vi "Main.vi"() -> ()   [LabVIEW 2021]
uses:
  DAQmxParams.ctl
  <vilib>/DAQmx/write.llb/DAQmx Write (Analog Wfm 1Chan NSamp).vi
  <vilib>/DAQmx/read.llb/DAQmx Read (Analog 1D Wfm NChan NSamp).vi
  <vilib>/DAQmx/create/channels.llb/DAQmx Create Channel (AO-Voltage-Basic).vi
  <vilib>/measure/matone.llb/Extract Single Tone Information 1 Chan.vi
  <vilib>/DAQmx/configure/timing.llb/DAQmx Timing (Sample Clock).vi
  <vilib>/DAQmx/miscellaneous.llb/DAQmx Fill In Error Info.vi
  <vilib>/DAQmx/create/channels.llb/DAQmx Create Channel (AI-Voltage-Basic).vi
  <vilib>/DAQmx/configure/trigger.llb/DAQmx Start Trigger (Analog Edge).vi
  <vilib>/measure/matone.llb/Extract Single Tone Information N Chan.vi
  <vilib>/measure/NI_MABase.lvlib
  <vilib>/measure/NI_MAPro.lvlib
panel:
  in  "Folder Path":path
  in  "Interval (ms)":dbl
  in  "Analyze Frequency":bool
  in  "Save analisys to file":bool
  in  "Stop frequency (Hz)":dbl
  in  "Start frequency (Hz)":dbl
  out "Phase":T1(graph)
  out "Amplitude":T2(graph)
  in  "Simulation":bool
  in  "V_out channel":tag
  in  "N samples/write":i32(slide)=1 min=1 scale=0.0..1000.0
  in  "Samples/s":i32=1 min=1
  in  "Trigger Channel":string(combo)
  in  "Function gen. 2":bool
  in  "Function gen. 1":bool
  in  "Frequency 2 (Hz)":dbl(knob) scale=0.0..10000.0
  in  "Amplitude 2 (V)":dbl(slide) scale=0.0..10.0
  in  "Frequency 1 (Hz)":dbl(knob) scale=0.0..10000.0
  in  "Amplitude 1 (V)":dbl(slide) scale=0.0..10.0
  in  "V_W Aq":bool
  in  "V_T Aq":bool
  in  "V_S Aq":bool
  in  "V_W":tag
  in  "V_T":tag
  in  "V_S":tag
  in  "Save acquisition to file":bool
  in  "DAQ Params":T3 {"Trigger Slope" items=["Rising"=10280, "Falling"=10171, "None"=0]; "Trigger Level" scale=-10.0..10.0}
  in  "Acquisition":bool
  out "Acquisition graph":waveform(dbl)[](graph)
  # "Function generator"
  # "Data acquisition"
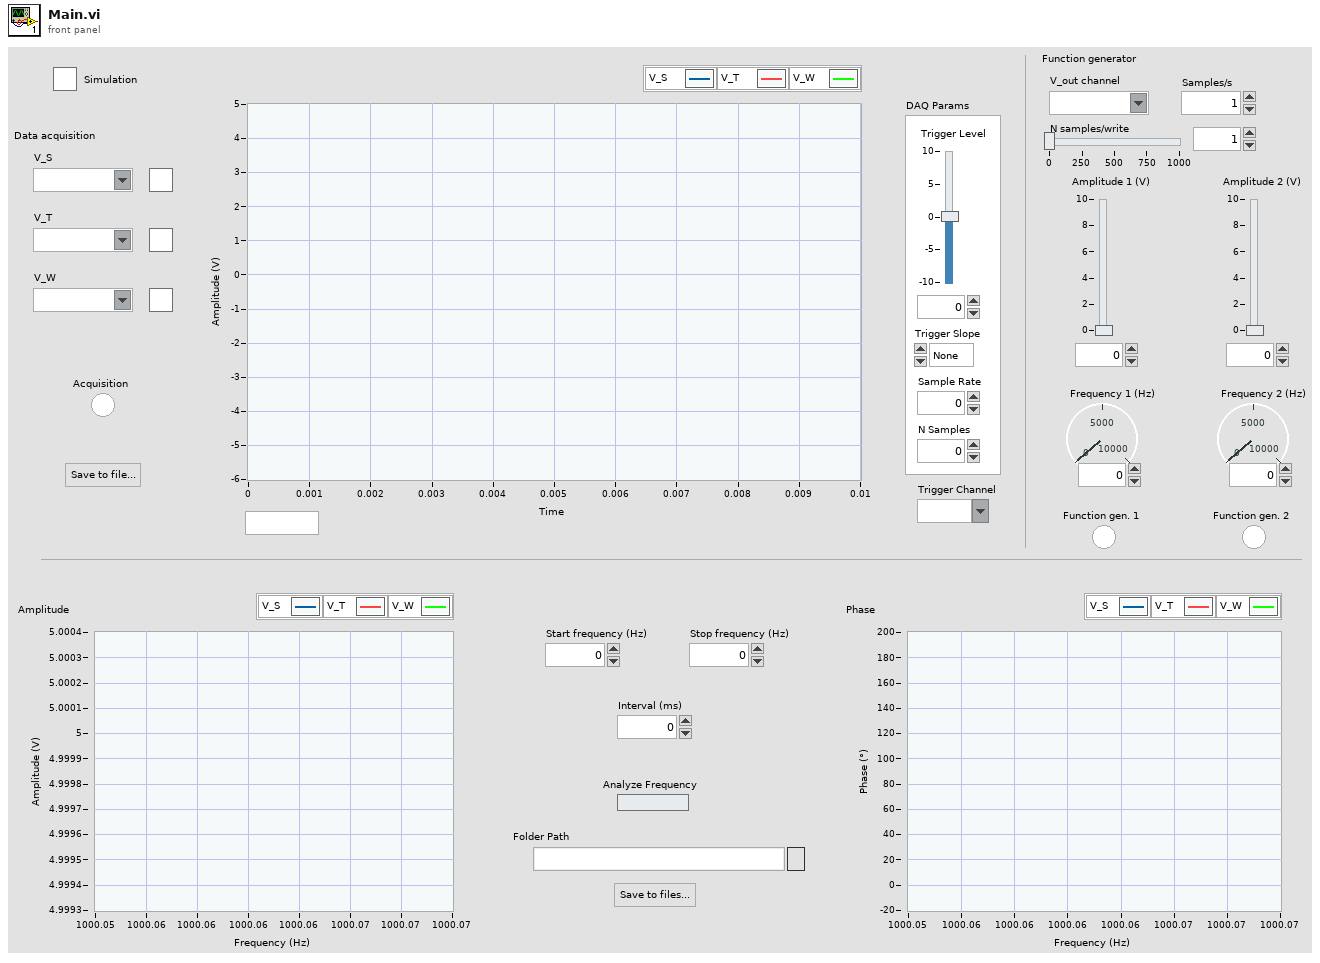
[diagram p1: front panel]
types:
  T1 = cluster{"detected frequencies":dbl[], "detected phases (deg)":dbl[]}[]
  T2 = cluster{"detected frequencies":dbl[], "detected amplitudes":dbl[]}[]
  T3 = typedef "DAQmxParams.ctl" = cluster{"Trigger Level":dbl, "Trigger Slope":i32, "Sample Rate":dbl, "N Samples":i32}
  T4 = enum8{"Enabled", "Disabled", "Disabled and Grayed Out"}
  T5 = enum16{"Sine Wave", "Triangle Wave", "Square Wave", "Sawtooth Wave"}
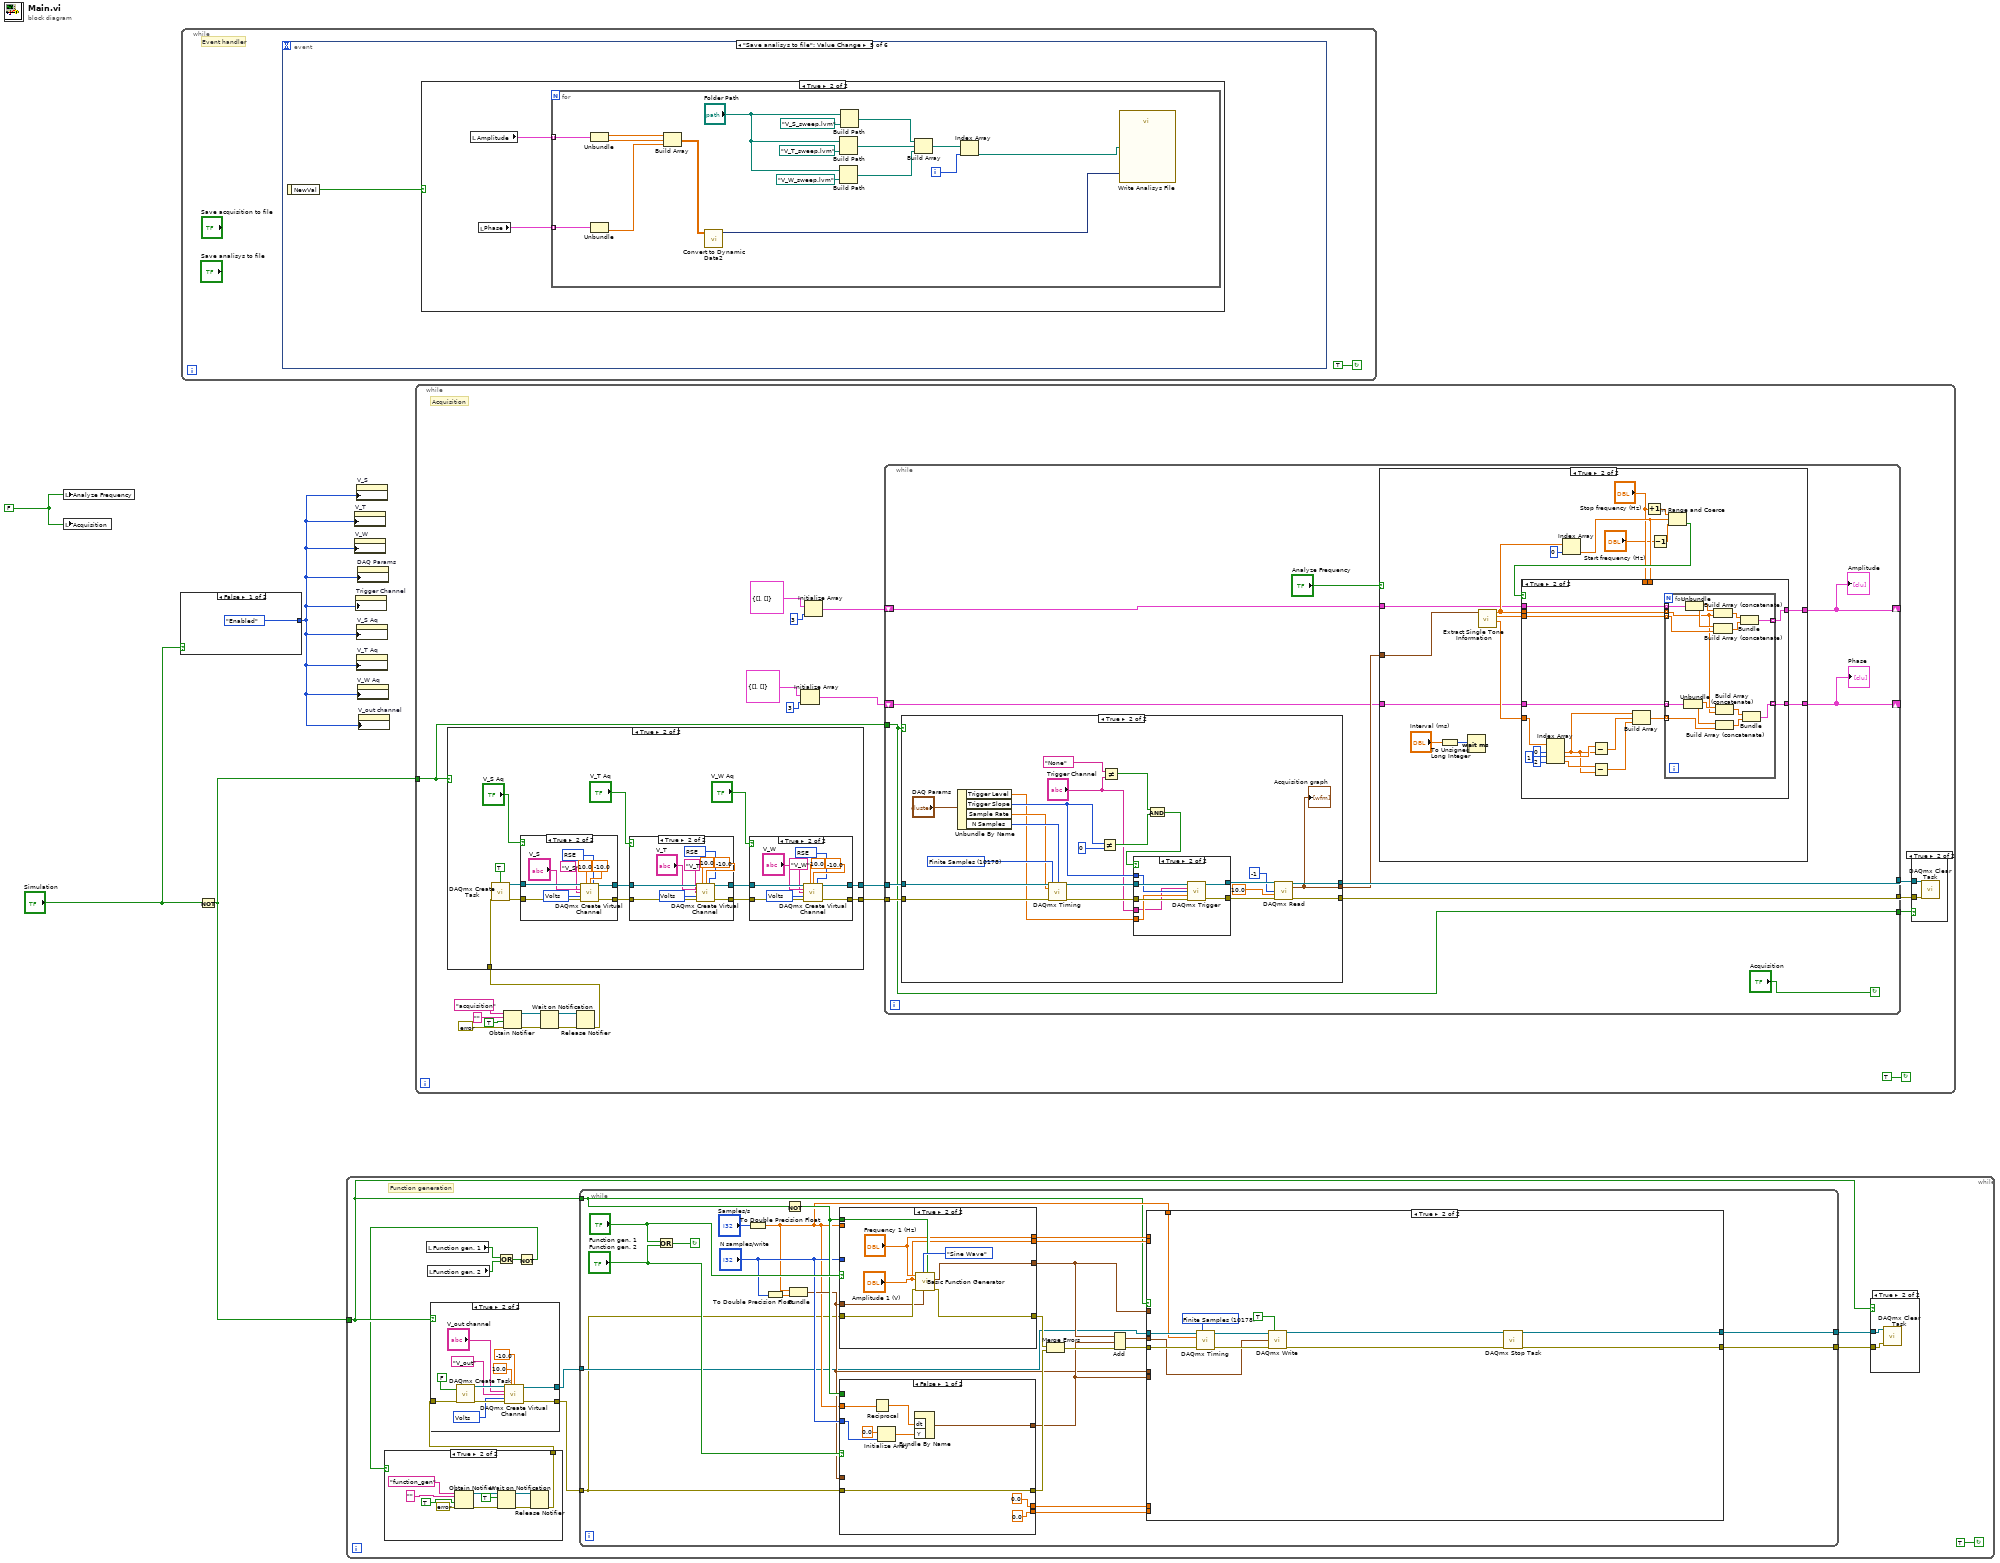
[diagram p0: block diagram]
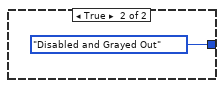
[diagram p2: hidden frame]
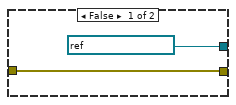
[diagram p4: hidden frame]
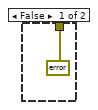
[diagram p5: hidden frame]
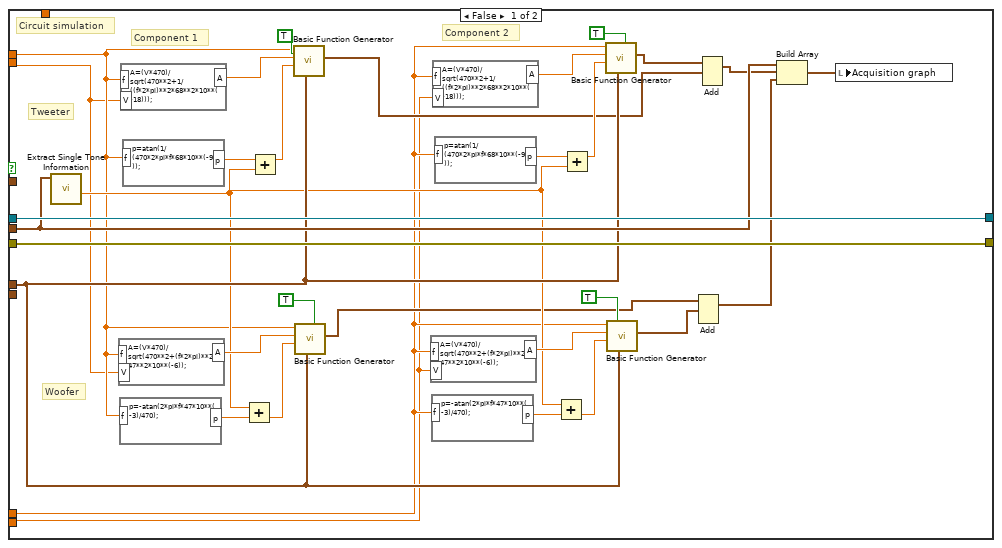
[diagram p6: hidden frame]
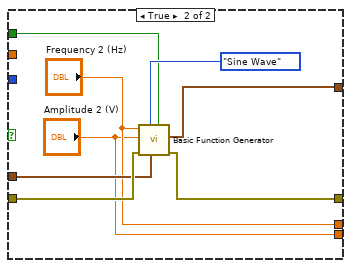
[diagram p7: hidden frame]
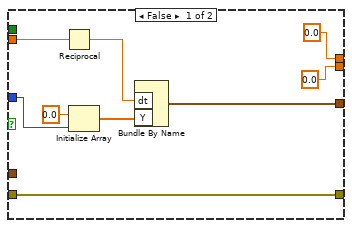
[diagram p8: hidden frame]
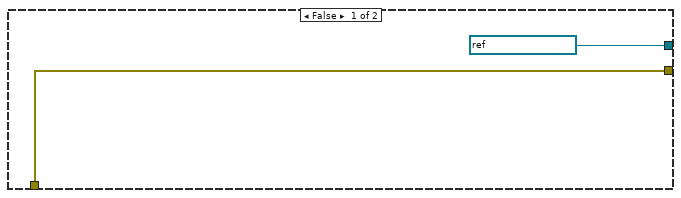
[diagram p10: hidden frame]
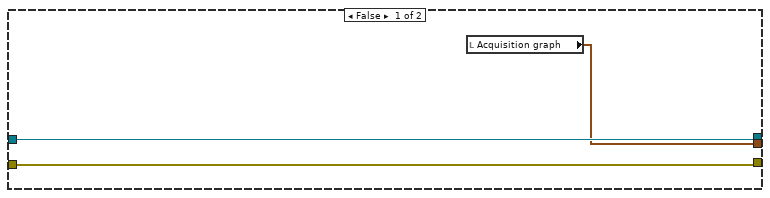
[diagram p14: hidden frame]
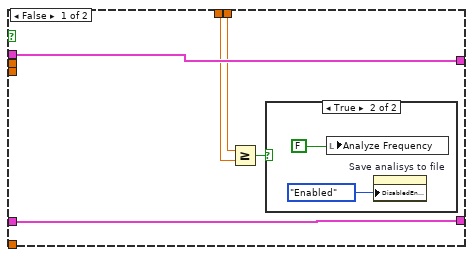
[diagram p17: hidden frame]
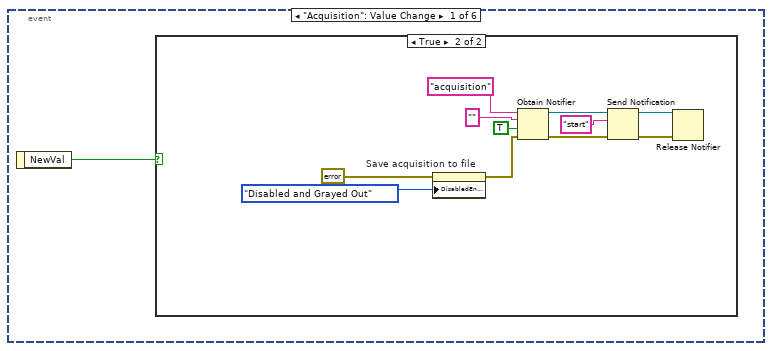
[diagram p19: hidden frame]
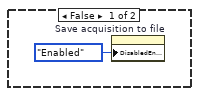
[diagram p20: hidden frame]
diagram:
  w1 = FALSE ("Acquisition")
  n1 = local write "Analyze Frequency"(w1) -> ()
  n2 = local write "Acquisition"(w1) -> ()
  n3 = case shown="False" "Simulation" {
    tunnel: [T4."Enabled" ("Disabled") T4."Disabled and Grayed Out" ("Disabled")] -> w2
    frame False {
    }
    frame True {
    }
  }
  n4 = while {
    stop <- TRUE continue-if-true
    # "Event handler"
    n5 = event shown="[4] \"Save analisys to file\": Value Change" {
      selector: _ -> [_ _ _ _ _ _]
      dyn-events: _ -> [_ _ _ _ _ _]
      timeout: _ -> [_ _ _ _ _ _]
      event "Acquisition": Value Change {
        n6 = event-data() -> ("NewVal"=w8:bool)  [unwired: 1 in]
        n7 = case shown="True" w8 {
          frame False {
            n8 = property on="Save acquisition to file" class="Bool"("DisabledEnum"=T4."Enabled" ("Disabled")) -> ()  [unwired: 2 in, 2 out]
          }
          frame True {
            n9 = property on="Save acquisition to file" class="Bool"(error in=errorcluster {"status"=FALSE, "code"=0, "source"=""} ("error in (no error)"), "DisabledEnum"=T4."Disabled and Grayed Out" ("Disabled")) -> (error out=w19:errorcluster)  [unwired: 1 in, 1 out]
            n10 = Obtain Notifier(name (unnamed)="acquisition", notification data type="" ("notification"), create if not found? (T)=TRUE, error in (no error)=w19) -> (notifier out=w16:refnum<notifier>, error out=w17:errorcluster)  [unwired: 1 out]
            n11 = Send Notification(notification="start", notifier=w16, error in (no error)=w17) -> (notifier out=w14:refnum<notifier>, error out=w13:errorcluster)
            n12 = Release Notifier(notifier=w14, error in (no error)=w13) -> ()  [unwired: 1 in, 3 out]
          }
        }
      }
      event "Save acquisition to file": Value Change {
        n13 = event-data() -> ("NewVal"=w21:bool)  [unwired: 1 in]
        n14 = case shown="True" w21 {
          frame False {
          }
          frame True {
            n15 = local read "Acquisition graph"() -> (w23:waveform(dbl)[])
            n16 = call "Convert to Dynamic Data"("Array of Waveforms"=w23) -> ("Dynamic Data Type"=w22:dynamicdata)  [unwired: 3 in]
            n17 = call "Write To Measurement File"("Signals"=w22) -> ()  [unwired: 16 in, 3 out]
          }
        }
      }
      event "Function gen. 1": Value Change {
        n18 = event-data() -> ("NewVal"=w24:bool)  [unwired: 1 in]
        n19 = case shown="True" w24 {
          frame False {
          }
          frame True {
            n20 = Obtain Notifier(name (unnamed)="function_gen", notification data type="" ("name (unnamed)"), create if not found? (T)=TRUE, error in (no error)=errorcluster {"status"=FALSE, "code"=0, "source"=""}) -> (notifier out=w29:refnum<notifier>, error out=w27:errorcluster)  [unwired: 1 out]
            n21 = Send Notification(notification="start", notifier=w29, error in (no error)=w27) -> (notifier out=w26:refnum<notifier>, error out=w25:errorcluster)
            n22 = Release Notifier(notifier=w26, error in (no error)=w25) -> ()  [unwired: 1 in, 3 out]
          }
        }
      }
      event "Function gen. 2": Value Change {
        n23 = event-data() -> ("NewVal"=w34:bool)  [unwired: 1 in]
        n24 = case shown="True" w34 {
          frame False {
          }
          frame True {
            n25 = Obtain Notifier(name (unnamed)="function_gen", notification data type="" ("name (unnamed)"), create if not found? (T)=TRUE, error in (no error)=errorcluster {"status"=FALSE, "code"=0, "source"=""}) -> (notifier out=w39:refnum<notifier>, error out=w37:errorcluster)  [unwired: 1 out]
            n26 = Send Notification(notification="start", notifier=w39, error in (no error)=w37) -> (notifier out=w36:refnum<notifier>, error out=w35:errorcluster)
            n27 = Release Notifier(notifier=w36, error in (no error)=w35) -> ()  [unwired: 1 in, 3 out]
          }
        }
      }
      event "Save analisys to file": Value Change {
        n28 = event-data() -> ("NewVal"=w44:bool)  [unwired: 1 in]
        n29 = case shown="True" w44 {
          frame False {
          }
          frame True {
            n30 = local read "Amplitude"() -> (w46:T2)
            n31 = local read "Phase"() -> (w45:T1)
            n32 = for {
              tunnel: w46 -> [w63] mode=indexing
              tunnel: w45 -> [w60] mode=indexing
              i -> [w48]
              n33 = Unbundle(w63) -> ("detected frequencies"=w62:dbl[], "detected amplitudes"=w61:dbl[])
              n34 = Unbundle(w60) -> ("detected phases (deg)"=w59:dbl[])  [unwired: 1 out]
              n35 = Build Array(w62, w61, w59) -> (w58:dbl[][])
              n36 = call "Convert to Dynamic Data2"("2D Array"=w58) -> ("Dynamic Data Type"=w57:dynamicdata)  [unwired: 3 in]
              n37 = Build Path(base path="Folder Path", name or relative path=path "V_T_sweep.lvm") -> (appended path=w51:path)
              n38 = Build Path(base path="Folder Path", name or relative path=path "V_W_sweep.lvm") -> (appended path=w50:path)
              n39 = Build Path(base path="Folder Path", name or relative path=path "V_S_sweep.lvm") -> (appended path=w52:path)
              n40 = Build Array(w52, w51, w50) -> (w49:path[])
              n41 = Index Array(array=w49, index=w48) -> (element=w47:path)
              n42 = call "Write Analisys File"("Signals"=w57, "Filename"=w47) -> ()  [unwired: 15 in, 3 out]
            }
          }
        }
      }
      event "Analyze Frequency": Value Change {
        n43 = event-data() -> ("NewVal"=w64:bool)  [unwired: 1 in]
        n44 = case shown="False" w64 {
          frame False {
            n45 = property on="Save analisys to file" class="Bool"("DisabledEnum"=T4."Enabled" ("Disabled")) -> ()  [unwired: 2 in, 2 out]
          }
          frame True {
            n46 = property on="Save analisys to file" class="Bool"("DisabledEnum"=T4."Disabled and Grayed Out" ("Disabled")) -> ()  [unwired: 2 in, 2 out]
          }
        }
      }
    }
  }
  n47 = Not(x="Simulation") -> (.not. x?=w4:bool)
  n48 = while {
    tunnel: w4 -> [w76]
    stop <- TRUE continue-if-true
    # "Function generation"
    n49 = local read "Function gen. 1"() -> (w72:bool)
    n50 = local read "Function gen. 2"() -> (w73:bool)
    n51 = Or(x=w72, y=w73) -> (x .or. y?=w74:bool)
    n52 = Not(x=w74) -> (.not. x?=w75:bool)
    n53 = case shown="True" w75 {
      tunnel: [errorcluster {"status"=FALSE, "code"=0, "source"=""} ("error out") w94] -> w71
      frame False {
      }
      frame True {
        n54 = Obtain Notifier(name (unnamed)="function_gen", notification data type="" ("name (unnamed)"), create if not found? (T)=TRUE, error in (no error)=errorcluster {"status"=FALSE, "code"=0, "source"=""}) -> (notifier out=w100:refnum<notifier>, error out=w101:errorcluster)  [unwired: 1 out]
        n55 = Wait on Notification(notifier=w100, ignore previous (F)=TRUE, error in (no error)=w101) -> (notifier out=w102:refnum<notifier>, error out=w103:errorcluster)  [unwired: 1 in, 2 out]
        n56 = Release Notifier(notifier=w102, error in (no error)=w103) -> (error out=w94:errorcluster)  [unwired: 1 in, 2 out]
      }
    }
    n57 = case shown="True" w76 {
      tunnel: w71 -> [w81 w92]
      tunnel: [refnum<k21> "DAQ Voltage_0" ("task out") w84] -> w70
      tunnel: [w81 w83] -> w69
      frame False {
      }
      frame True {
        w86 = 10348 items=["Volts"=10348, "From Custom Scale"=10065] ("units")
        n58 = call <vilib>:"DAQmx Create Task.vi"("auto cleanup"=FALSE, "error in"=w92) -> ("task out"=w88:refnum<k21>, "error out"=w87:errorcluster)  [unwired: 12 in]
        n59 = call-poly <vilib>:"DAQmx Create Virtual Channel.vi"("task in"=w88, "maximum value"=10.0, "minimum value"=-10.0, "physical channels"="V_out channel", "name to assign"="V_out", "units"=w86, "error in"=w87) -> ("task out"=w84:refnum<k21>, "error out"=w83:errorcluster)  [unwired: 7 in]
      }
    }
    n60 = while {
      tunnel: w76 -> [w108]
      tunnel: w70 -> [w107]
      tunnel: w69 -> [w106]
      tunnel: [w105] -> w68
      tunnel: [w104] -> w67
      stop <- w122 continue-if-true
      n61 = Or(x="Function gen. 1", y="Function gen. 2") -> (x .or. y?=w122:bool)
      n62 = To Double Precision Float(number="Samples/s") -> (double precision float=w109:dbl)
      n63 = To Double Precision Float(number="N samples/write") -> (double precision float=w116:dbl)
      n64 = Not(x=w108) -> (.not. x?=w117:bool)
      n65 = Bundle(w109, w116) -> (w114:cluster{dbl, dbl})  [unwired: 1 in]
      n66 = case shown="True" "Function gen. 1" {
        tunnel: [w196 w204] -> w119
        tunnel: "N samples/write" -> [w195 _]
        tunnel: [w192 w205] -> w126
        tunnel: w109 -> [w193 _]
        tunnel: w106 -> [w192 w203]
        tunnel: w117 -> [_ w202]
        tunnel: w114 -> [_ w201]
        tunnel: [0.0 ("Frequency 1 (Hz)") "Frequency 1 (Hz)"] -> w113
        tunnel: [0.0 ("Amplitude 1 (V)") "Amplitude 1 (V)"] -> w111
        frame False {
          n67 = Reciprocal(x=w193) -> (1/x=w194:dbl)
          n68 = Initialize Array(0.0 ("element"), w195) -> (w197:dbl[])
          n69 = Bundle By Name("dt"=w194, "Y"=w197) -> (w196:waveform(dbl))  [unwired: 1 in]
        }
        frame True {
          n70 = call <vilib>:"Basic Function Generator.vi"("reset signal"=w202, "sampling info"=w201, "signal type"=T5."Sine Wave", "error in (no error)"=w203, "amplitude"="Amplitude 1 (V)", "frequency"="Frequency 1 (Hz)") -> ("error out"=w205:errorcluster, "signal out"=w204:waveform(dbl))  [unwired: 3 in, 1 out]
        }
      }
      n71 = case shown="False" "Function gen. 2" {
        tunnel: [w181 w187] -> w118
        tunnel: "N samples/write" -> [w178 _]
        tunnel: [w175 w189] -> w125
        tunnel: w109 -> [w176 _]
        tunnel: w106 -> [w175 w186]
        tunnel: w117 -> [_ w185]
        tunnel: w114 -> [_ w184]
        tunnel: [0.0 ("Frequency 2 (Hz)") "Frequency 2 (Hz)"] -> w112
        tunnel: [0.0 ("Amplitude 2 (V)") "Amplitude 2 (V)"] -> w110
        frame False {
          n72 = Reciprocal(x=w176) -> (1/x=w177:dbl)
          n73 = Initialize Array(0.0 ("element"), w178) -> (w179:dbl[])
          n74 = Bundle By Name("dt"=w177, "Y"=w179) -> (w181:waveform(dbl))  [unwired: 1 in]
        }
        frame True {
          n75 = call <vilib>:"Basic Function Generator.vi"("reset signal"=w185, "sampling info"=w184, "signal type"=T5."Sine Wave", "error in (no error)"=w186, "amplitude"="Amplitude 2 (V)", "frequency"="Frequency 2 (Hz)") -> ("error out"=w189:errorcluster, "signal out"=w187:waveform(dbl))  [unwired: 3 in, 1 out]
        }
      }
      n76 = Merge Errors(w126, w125) -> (w124:errorcluster)
      n77 = Add(1:w118, 2:w119, 4:w124) -> (0:w120:waveform(dbl), 3:w121:errorcluster)
      n78 = case shown="True" w108 {
        tunnel: w121 -> [w159 w169]
        tunnel: w107 -> [w160 w168]
        tunnel: [w159 w161] -> w104
        tunnel: [w160 w162] -> w105
        tunnel: w120 -> [w155 w167]
        tunnel: w119 -> [_ _]
        tunnel: w118 -> [_ _]
        tunnel: w114 -> [w141 _]
        tunnel: w113 -> [w133 _]
        tunnel: w112 -> [w132 _]
        tunnel: w111 -> [w131 _]
        tunnel: w110 -> [w130 _]
        tunnel: w109 -> [_ w166]
        frame False {
          # "Woofer"
          # "Tweeter"
          # "Component 2"
          # "Component 1"
          # "Circuit simulation"
          n79 = call-poly <vilib>:"Extract Single Tone Information.vi"("time signal in"=w155) -> ("detected phase (deg)"=w140:dbl)  [unwired: 5 in, 5 out]
          n80 = formula code="A=(V*470)/sqrt(470**2+(f*2*pi)**2*47**2*10**(-6));"("f"=w133, "V"=w131) -> ("A"=w156:dbl)
          n81 = formula code="p=-atan(2*pi*f*47*10**(-3)/470);"("f"=w133) -> ("p"=w152:dbl)
          n82 = formula code="A=(V*470)/sqrt(470**2+1/((f*2*pi)**2*68**2*10**(-18)));"("f"=w133, "V"=w131) -> ("A"=w157:dbl)
          n83 = formula code="p=atan(1/(470*2*pi*f*68*10**(-9)));"("f"=w133) -> ("p"=w154:dbl)
          n84 = Add(x=w140, y=w152) -> (x+y=w149:dbl)
          n85 = Add(x=w154, y=w140) -> (x+y=w150:dbl)
          n86 = call <vilib>:"Basic Function Generator.vi"("reset signal"=TRUE, "sampling info"=w141, "phase"=w150, "amplitude"=w157, "frequency"=w133) -> ("signal out"=w138:waveform(dbl))  [unwired: 4 in, 2 out]
          n87 = call <vilib>:"Basic Function Generator.vi"("reset signal"=TRUE, "sampling info"=w141, "phase"=w149, "amplitude"=w156, "frequency"=w133) -> ("signal out"=w135:waveform(dbl))  [unwired: 4 in, 2 out]
          n88 = formula code="A=(V*470)/sqrt(470**2+(f*2*pi)**2*47**2*10**(-6));"("f"=w132, "V"=w130) -> ("A"=w147:dbl)
          n89 = formula code="p=-atan(2*pi*f*47*10**(-3)/470);"("f"=w132) -> ("p"=w145:dbl)
          n90 = formula code="A=(V*470)/sqrt(470**2+1/((f*2*pi)**2*68**2*10**(-18)));"("f"=w132, "V"=w130) -> ("A"=w148:dbl)
          n91 = formula code="p=atan(1/(470*2*pi*f*68*10**(-9)));"("f"=w132) -> ("p"=w146:dbl)
          n92 = Add(x=w140, y=w145) -> (x+y=w142:dbl)
          n93 = Add(x=w146, y=w140) -> (x+y=w143:dbl)
          n94 = call <vilib>:"Basic Function Generator.vi"("reset signal"=TRUE, "sampling info"=w141, "phase"=w143, "amplitude"=w148, "frequency"=w132) -> ("signal out"=w139:waveform(dbl))  [unwired: 4 in, 2 out]
          n95 = call <vilib>:"Basic Function Generator.vi"("reset signal"=TRUE, "sampling info"=w141, "phase"=w142, "amplitude"=w147, "frequency"=w132) -> ("signal out"=w136:waveform(dbl))  [unwired: 4 in, 2 out]
          n96 = Add(1:w136, 2:w135) -> (0:w134:waveform(dbl))  [unwired: 1 in, 1 out]
          n97 = Add(1:w138, 2:w139) -> (0:w137:waveform(dbl))  [unwired: 1 in, 1 out]
          n98 = Build Array(w155, w137, w134) -> (w158:waveform(dbl)[])
          n99 = local write "Acquisition graph"(w158) -> ()
        }
        frame True {
          w172 = 10178 items=["Finite Samples"=10178, "Continuous Samples"=10123, "Hardware Timed Single Point"=12522] ("sample mode")
          n100 = call-poly <vilib>:"DAQmx Timing.vi"("task/channels in"=w168, "sample mode"=w172, "rate"=w166, "error in"=w169) -> ("task out"=w171:refnum<k21>, "error out"=w170:errorcluster)  [unwired: 10 in]
          n101 = call-poly <vilib>:"DAQmx Write.vi"("task/channels in"=w171, "auto start"=TRUE, "data"=w167, "error in"=w170) -> ("task out"=w164:refnum<k21>, "error out"=w163:errorcluster)  [unwired: 9 in, 1 out]
          n102 = call <vilib>:"DAQmx Stop Task.vi"("task/channels in"=w164, "error in"=w163) -> ("task out"=w162:refnum<k21>, "error out"=w161:errorcluster)  [unwired: 12 in]
        }
      }
    }
    n103 = case shown="True" w76 {
      tunnel: w68 -> [_ w79]
      tunnel: w67 -> [_ w78]
      frame False {
      }
      frame True {
        n104 = call <vilib>:"DAQmx Clear Task.vi"("task in"=w79, "error in"=w78) -> ()  [unwired: 13 in, 1 out]
      }
    }
  }
  n105 = property on="V_T" class="DAQmxName"("DisabledEnum"=w2) -> ()  [unwired: 2 in, 2 out]
  n106 = property on="V_W" class="DAQmxName"("DisabledEnum"=w2) -> ()  [unwired: 2 in, 2 out]
  n107 = property on="Trigger Channel" class="CmbBox"("DisabledEnum"=w2) -> ()  [unwired: 2 in, 2 out]
  n108 = property on="V_S" class="DAQmxName"("DisabledEnum"=w2) -> ()  [unwired: 2 in, 2 out]
  n109 = property on="V_S Aq" class="Bool (strict)"("DisabledEnum"=w2) -> ()  [unwired: 2 in, 2 out]
  n110 = property on="V_T Aq" class="Bool (strict)"("DisabledEnum"=w2) -> ()  [unwired: 2 in, 2 out]
  n111 = property on="DAQ Params" class="Clust (strict)"("DisabledEnum"=w2) -> ()  [unwired: 2 in, 2 out]
  n112 = property on="V_W Aq" class="Bool (strict)"("DisabledEnum"=w2) -> ()  [unwired: 2 in, 2 out]
  n113 = property on="V_out channel" class="DAQmxName"("DisabledEnum"=w2) -> ()  [unwired: 2 in, 2 out]
  n114 = while {
    tunnel: w4 -> [w214]
    stop <- TRUE continue-if-true
    # "Acquisition"
    n115 = Obtain Notifier(name (unnamed)="acquisition", notification data type="" ("notification"), create if not found? (T)=TRUE, error in (no error)=errorcluster {"status"=FALSE, "code"=0, "source"=""}) -> (notifier out=w226:refnum<notifier>, error out=w225:errorcluster)  [unwired: 1 out]
    n116 = Wait on Notification(notifier=w226, error in (no error)=w225) -> (notifier out=w223:refnum<notifier>, error out=w224:errorcluster)  [unwired: 2 in, 2 out]
    n117 = Release Notifier(notifier=w223, error in (no error)=w224) -> (error out=w222:errorcluster)  [unwired: 1 in, 2 out]
    n118 = case shown="True" w214 {
      tunnel: w222 -> [w232 w245]
      tunnel: [w232 w234] -> w219
      tunnel: [refnum<k21> "DAQ Voltage_0" ("task out") w233] -> w218
      frame False {
      }
      frame True {
        n119 = call <vilib>:"DAQmx Create Task.vi"("auto cleanup"=TRUE, "error in"=w245) -> ("task out"=w242:refnum<k21>, "error out"=w243:errorcluster)  [unwired: 12 in]
        n120 = case shown="True" "V_S Aq" {
          tunnel: w243 -> [w270 w281]
          tunnel: w242 -> [w271 w280]
          tunnel: [w271 w277] -> w241
          tunnel: [w270 w276] -> w240
          frame False {
          }
          frame True {
            w272 = 10348 items=["Volts"=10348, "From Custom Scale"=10065] ("units")
            w273 = 10083 items=["Default"=-1, "RSE"=10083, "NRSE"=10078, "Differential"=10106, "Pseudodifferential"=12529] ("input terminal configuration")
            n121 = call-poly <vilib>:"DAQmx Create Virtual Channel.vi"("task in"=w280, "maximum value"=10.0, "minimum value"=-10.0 ("maximum value"), "input terminal configuration"=w273, "physical channels"="V_S", "name to assign"="V_S", "units"=w272, "error in"=w281) -> ("task out"=w277:refnum<k21>, "error out"=w276:errorcluster)  [unwired: 6 in]
          }
        }
        n122 = case shown="True" "V_T Aq" {
          tunnel: w241 -> [w259 w269]
          tunnel: w240 -> [w258 w268]
          tunnel: [w259 w265] -> w239
          tunnel: [w258 w264] -> w238
          frame False {
          }
          frame True {
            w260 = 10348 items=["Volts"=10348, "From Custom Scale"=10065] ("units")
            w261 = 10083 items=["Default"=-1, "RSE"=10083, "NRSE"=10078, "Differential"=10106, "Pseudodifferential"=12529] ("input terminal configuration")
            n123 = call-poly <vilib>:"DAQmx Create Virtual Channel.vi"("task in"=w269, "maximum value"=10.0, "minimum value"=-10.0 ("maximum value"), "input terminal configuration"=w261, "physical channels"="V_T", "name to assign"="V_T", "units"=w260, "error in"=w268) -> ("task out"=w265:refnum<k21>, "error out"=w264:errorcluster)  [unwired: 6 in]
          }
        }
        n124 = case shown="True" "V_W Aq" {
          tunnel: w239 -> [w246 w257]
          tunnel: w238 -> [w247 w256]
          tunnel: [w247 w249] -> w234
          tunnel: [w246 w248] -> w233
          frame False {
          }
          frame True {
            w250 = 10348 items=["Volts"=10348, "From Custom Scale"=10065] ("units")
            w251 = 10083 items=["Default"=-1, "RSE"=10083, "NRSE"=10078, "Differential"=10106, "Pseudodifferential"=12529] ("input terminal configuration")
            n125 = call-poly <vilib>:"DAQmx Create Virtual Channel.vi"("task in"=w257, "maximum value"=10.0, "minimum value"=-10.0 ("maximum value"), "input terminal configuration"=w251, "physical channels"="V_W", "name to assign"="V_W", "units"=w250, "error in"=w256) -> ("task out"=w248:refnum<k21>, "error out"=w249:errorcluster)  [unwired: 6 in]
          }
        }
      }
    }
    n126 = Initialize Array(cluster{dbl[], dbl[]} {[], []}, 3 ("dimension size")) -> (w207:cluster{dbl[], dbl[]}[])
    n127 = Initialize Array(cluster{dbl[], dbl[]} {[], []}, 3 ("dimension size")) -> (w210:cluster{dbl[], dbl[]}[])
    n128 = while {
      tunnel: w219 -> [w291]
      tunnel: w218 -> [w292]
      tunnel: [w290] -> w217
      tunnel: [w289] -> w216
      shift-right: [w285] -> _
      shift-left: w210 -> [w286]
      shift-right: [w283] -> _
      shift-left: w207 -> [w284]
      tunnel: w214 -> [w282]
      tunnel: [w282] -> w213
      stop <- "Acquisition" continue-if-true
      n129 = case shown="True" w282 {
        tunnel: w292 -> [w296 w319]
        tunnel: w291 -> [w295 w318]
        tunnel: [w296 w299] -> w290
        tunnel: [w295 w298] -> w289
        tunnel: [w294 w297] -> w287
        frame False {
          n130 = local read "Acquisition graph"() -> (w294:waveform(dbl)[])
        }
        frame True {
          w315 = 10178 items=["Finite Samples"=10178, "Continuous Samples"=10123, "Hardware Timed Single Point"=12522] ("sample mode")
          n131 = Unbundle By Name("DAQ Params") -> ("Trigger Level"=w304:dbl, "Trigger Slope"=w308:i32, "Sample Rate"=w314:dbl, "N Samples"=w316:i32)
          n132 = call-poly <vilib>:"DAQmx Timing.vi"("task/channels in"=w319, "sample mode"=w315, "samples per channel"=w316, "rate"=w314, "error in"=w318) -> ("task out"=w310:refnum<k21>, "error out"=w309:errorcluster)  [unwired: 9 in]
          n133 = Not Equal?(x=w308, y=0) -> (x != y?=w312:bool)
          n134 = Not Equal?(x="None" ("Trigger Channel"), y="Trigger Channel") -> (x != y?=w306:bool)
          n135 = And(x=w306, y=w312) -> (x .and. y?=w311:bool)
          n136 = case shown="True" w311 {
            tunnel: w310 -> [w321 w328]
            tunnel: w309 -> [w320 w327]
            tunnel: w308 -> [_ w325]
            tunnel: "Trigger Channel" -> [_ w324]
            tunnel: w304 -> [_ w326]
            tunnel: [w321 w323] -> w303
            tunnel: [w320 w322] -> w302
            frame False {
            }
            frame True {
              n137 = call-poly <vilib>:"DAQmx Trigger.vi"("task/channels in"=w328, "source"=w324, "slope"=w325, "level"=w326, "error in"=w327) -> ("task out"=w323:refnum<k21>, "error out"=w322:errorcluster)  [unwired: 9 in]
            }
          }
          n138 = call-poly <vilib>:"DAQmx Read.vi"("task/channels in"=w303, "number of samples per channel"=-1, "timeout"=10.0, "error in"=w302) -> ("task out"=w299:refnum<k21>, "data"=w297:waveform(dbl)[], "error out"=w298:errorcluster)  [unwired: 9 in]
          "Acquisition graph" <- w297
        }
      }
      n139 = case shown="True" "Analyze Frequency" {
        tunnel: w287 -> [_ w346]
        tunnel: [w330 w343] -> w285
        tunnel: w286 -> [w330 w342]
        tunnel: [w329 w339] -> w283
        tunnel: w284 -> [w329 w338]
        frame False {
        }
        frame True {
          n140 = To Unsigned Long Integer(number="Interval (ms)") -> (unsigned 32bit integer=w334:u32)
          n141 = Wait (ms)(milliseconds to wait=w334) -> ()  [unwired: 1 out]
          n142 = call-poly <vilib>:"Extract Single Tone Information.vi"("time signals in"=w346) -> ("detected phases (deg)"=w340:dbl[], "detected amplitudes"=w341:dbl[], "detected frequencies"=w344:dbl[])  [unwired: 5 in, 3 out]
          n143 = Index Array(array=w344, index=0) -> (element=w337:dbl)
          n144 = Increment(x="Stop frequency (Hz)") -> (x+1=w331:dbl)
          n145 = Decrement(x="Start frequency (Hz)") -> (x-1=w332:dbl)
          n146 = In Range and Coerce(upper limit=w331, x=w337, lower limit=w332) -> (In Range?=w345:bool)  [unwired: 1 out]
          n147 = case shown="True" w345 {
            tunnel: w344 -> [_ w370]
            tunnel: [w352 w366] -> w343
            tunnel: w342 -> [w352 w368]
            tunnel: w341 -> [_ w369]
            tunnel: w340 -> [_ w361]
            tunnel: [w351 w365] -> w339
            tunnel: w338 -> [w351 w367]
            tunnel: w337 -> [w349 _]
            tunnel: "Stop frequency (Hz)" -> [w348 _]
            frame False {
              n148 = Greater Or Equal?(x=w349, y=w348) -> (x >= y?=w350:bool)
              n149 = case shown="True" w350 {
                frame False {
                }
                frame True {
                  n150 = local write "Analyze Frequency"(FALSE ("Analyze Frequency")) -> ()
                  n151 = property on="Save analisys to file" class="Bool"("DisabledEnum"=T4."Enabled" ("Disabled")) -> ()  [unwired: 2 in, 2 out]
                }
              }
            }
            frame True {
              n152 = Index Array(array=w361, index #1=0 ("index"), index #2=1 ("index"), index #3=2 ("index")) -> (element #1=w355:dbl, element #2=w360:dbl, element #3=w359:dbl)
              n153 = Subtract(x=w360, y=w355) -> (x-y=w357:dbl)
              n154 = Subtract(x=w359, y=w355) -> (x-y=w356:dbl)
              n155 = Build Array(w355, w357, w356) -> (w358:dbl[])
              n156 = for {
                tunnel: w370 -> [w373] mode=indexing
                tunnel: w369 -> [w381] mode=indexing
                tunnel: w368 -> [w385] mode=indexing
                tunnel: w367 -> [w384] mode=indexing
                tunnel: w358 -> [w374] mode=indexing
                tunnel: [w372] -> w366 mode=indexing
                tunnel: [w371] -> w365 mode=indexing
                n157 = Unbundle(w384) -> (w376:dbl[], w375:dbl[])
                n158 = Unbundle(w385) -> (w383:dbl[], w382:dbl[])
                n159 = Build Array (concatenate)(w383, w373) -> (w380:dbl[])
                n160 = Build Array (concatenate)(w382, w381) -> (w379:dbl[])
                n161 = Build Array (concatenate)(w376, w373) -> (w378:dbl[])
                n162 = Build Array (concatenate)(w375, w374) -> (w377:dbl[])
                n163 = Bundle(w380, w379) -> (w372:cluster{dbl[], dbl[]})  [unwired: 1 in]
                n164 = Bundle(w378, w377) -> (w371:cluster{dbl[], dbl[]})  [unwired: 1 in]
              }
            }
          }
        }
      }
      "Amplitude" <- w285
      "Phase" <- w283
    }
    n165 = case shown="True" w213 {
      tunnel: w217 -> [_ w230]
      tunnel: w216 -> [_ w229]
      frame False {
      }
      frame True {
        n166 = call <vilib>:"DAQmx Clear Task.vi"("task in"=w230, "error in"=w229) -> ()  [unwired: 13 in, 1 out]
      }
    }
  }
